vi "popup timer.vi"(8 "error in (no error)":errorcluster, 10 "target time (sec)":dbl=30.0 format="%#_13g") -> (0 "error out":errorcluster)   [LabVIEW 2020]
panel:
  out "Countdown":dbl=1653.7379999160767 caption="seconds" format="%#_2g"
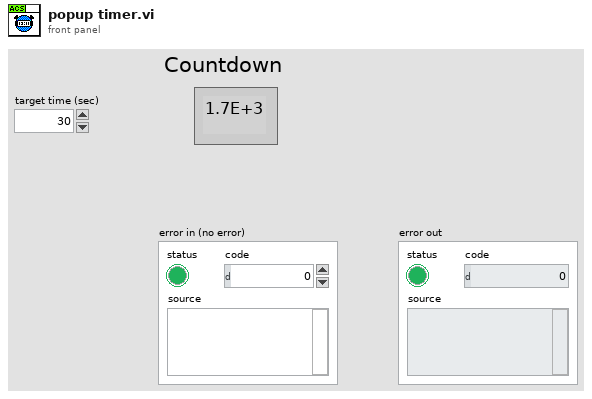
[diagram p1: front panel]
types:
  T1 = enum16{"Start Timer", "Get Time", "Pause", "Unpause"}
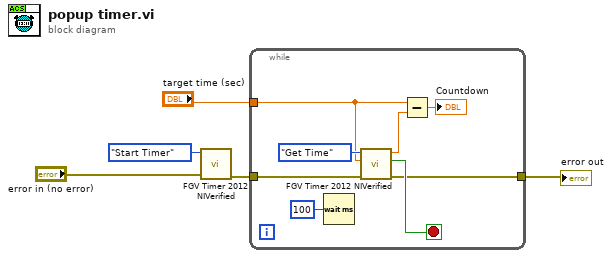
[diagram p0: block diagram]
diagram:
  n1 = call "FGV Timer 2012 NIVerified.vi"("error in (no error)"="error in (no error)", "Enum"=T1."Start Timer") -> ("error out"=w5:errorcluster)  [unwired: 6 in, 3 out]
  n2 = while {
    tunnel: w5 -> [w11]
    tunnel: [w10] -> w1
    tunnel: "target time (sec)" -> [w6]
    stop <- w12 stop-if-true
    n3 = Wait (ms)(milliseconds to wait=u32 100) -> ()  [unwired: 1 out]
    n4 = call "FGV Timer 2012 NIVerified.vi"("error in (no error)"=w11, "Target Time (sec)"=w6, "Enum"=T1."Get Time") -> ("error out"=w10:errorcluster, "Time Elapsed?"=w12:bool, "Elapsed Time"=w7:dbl)  [unwired: 5 in, 1 out]
    n5 = Subtract(x=w6, y=w7) -> (x-y=→"Countdown":dbl)
  }
  "error out" <- w1
